vi "Check Consistency.vi"(8 "error in":errorcluster, 11 "Plugin_Controller in":refnum<class "Plugin_Controller.lvclass">) -> (0 "error out":errorcluster, 1 "Result Messages":T1[](array[typedef]), 2 "Node OK":bool, 3 "Plugin_Controller out":refnum<class "Plugin_Controller.lvclass">)   [LabVIEW 2020, in "Plugin.lvlib" / "Plugin_Controller.lvclass"]
doc: "Checks if the Plugin's configuration is consistent for test execution."
uses:
  Plugin_Controller.lvclass
  C:/SVN_LabSys/labsys_lvcode/LabSys_SourceCode/builds/Libraries/LabSys Framework.lvlibp/Configurable Data Node/Configurable Data Node/Configurable Data Node.lvclass
  builds/Libraries/LabSys Framework.lvlibp/Data Node/Data Node/Result.ctl
  builds/Libraries/LabSys Framework.lvlibp/Data Node/Data Node/Result Type.ctl
  builds/Libraries/LabSys Framework.lvlibp/Configurable Data Node/Configurable Data Node/Read Module Configuration.vi
  builds/Libraries/LabSys Framework.lvlibp/Configuration Storage/Module Configuration/Module Configuration.lvclass
  builds/Libraries/LabSys Framework.lvlibp/Data Node/Data Node/Data Node.lvclass
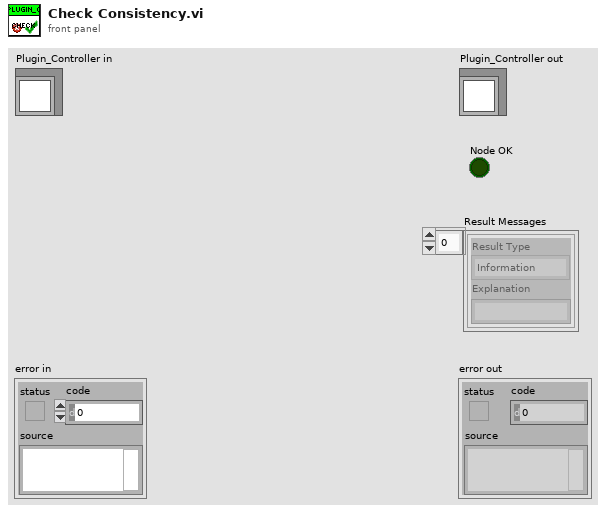
[diagram p1: front panel]
types:
  T1 = typedef "LabSys Framework.lvlibp/Data Node.lvlib/Data Node.lvclass/Result.ctl" = cluster{"Result Type":T2, "Explanation":string}
  T2 = typedef "LabSys Framework.lvlibp/Data Node.lvlib/Data Node.lvclass/Result Type.ctl" = enum16{"Information", "Warning", "Error"}
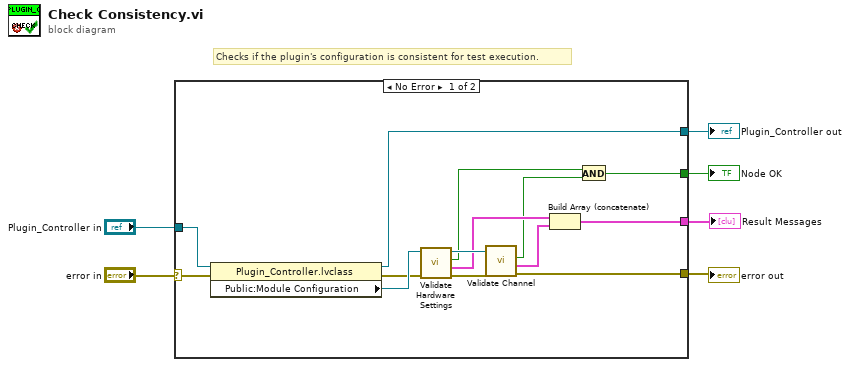
[diagram p0: block diagram]
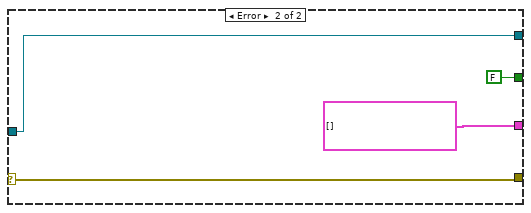
[diagram p2: hidden frame]
diagram:
  # "Checks if the plugin's configuration is consistent for test execution."
  n1 = case shown="No Error" "error in" {
    selector: "error in" -> [w20 w21]
    tunnel: "Plugin_Controller in" -> [w19 w24]
    tunnel: [w10 FALSE] -> w4
    tunnel: [w9 T1[] []] -> w3
    tunnel: [w8 w21] -> w2
    tunnel: [w7 w24] -> w1
    frame No Error {
      n2 = property class="Plugin_Controller.lvclass"(reference=w19, error in=w20) -> (reference out=w7:refnum<class "Plugin_Controller.lvclass">, error out=w17:errorcluster, "Public:Module Configuration"=w18:refnum<class "Module Configuration.lvclass">)
      n3 = call "Validate Hardware Settings.vi"("error in"=w17, "Module Configuration in"=w18) -> ("error out"=w16:errorcluster, "Result Messages"=w13:T1[], "Config OK"=w11:bool, "Module Configuration out"=w15:refnum<class "Module Configuration.lvclass">)  [unwired: 6 in]
      n4 = call "Validate Channel.vi"("error in"=w16, "Module Configuration"=w15) -> ("error out"=w8:errorcluster, "Result Messages"=w14:T1[], "Config OK"=w12:bool)  [unwired: 6 in, 1 out]
      n5 = Build Array (concatenate)(w13, w14) -> (w9:T1[])
      n6 = And(x=w11, y=w12) -> (x .and. y?=w10:bool)
    }
    frame Error {
    }
  }
  "error out" <- w2
  "Plugin_Controller out" <- w1
  "Node OK" <- w4
  "Result Messages" <- w3
